vi "读取缺试剂参数.vi"(0 "MB session in":refnum<class "MB_Master.lvclass">, 5 "error in (no error)":errorcluster) -> (14 "MB session out":refnum<class "MB_Master.lvclass">, 15 "评价结果":bool[](array[boolean]), 16 "CH光值":u16[](array[numeric]), 17 "缺试剂类型":u8[](array[numeric]), 18 "光强阈值":u16[](array[numeric]), 19 "error out":errorcluster)   [LabVIEW 2016, in "斯坦道CODMn新电路板.lvlib"]
uses:
  <vilib>/Plasmionique/MB Master/MB_Master/MB_Master.lvclass
  <vilib>/Plasmionique/MB Master/MB_Master_Serial/MB_Master_Serial.lvclass
  D:/Program Files (x86)/National Instruments/LabVIEW 2016/vi.lib/Plasmionique/MB Master/MB_Master/MB_Master.lvclass
  <vilib>/Plasmionique/MB Master/MB Master.lvlib
panel:
  in  "VISA Resource":refnum<visa-resource-name>
  in  "引用选择":enum16{"MB引用", "自建引用"}(ring)
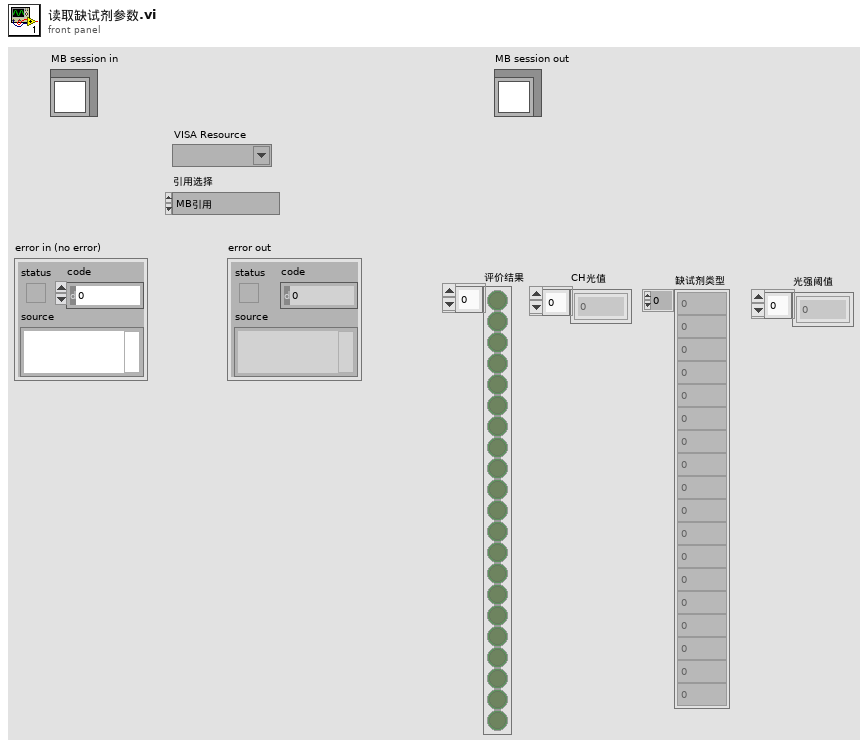
[diagram p1: front panel]
types:
  T1 = cluster{"baud rate (bps)":u32, "stop bits":u16, "parity":u16, "flow control":u16, "timeout":u32, "retries":i32}
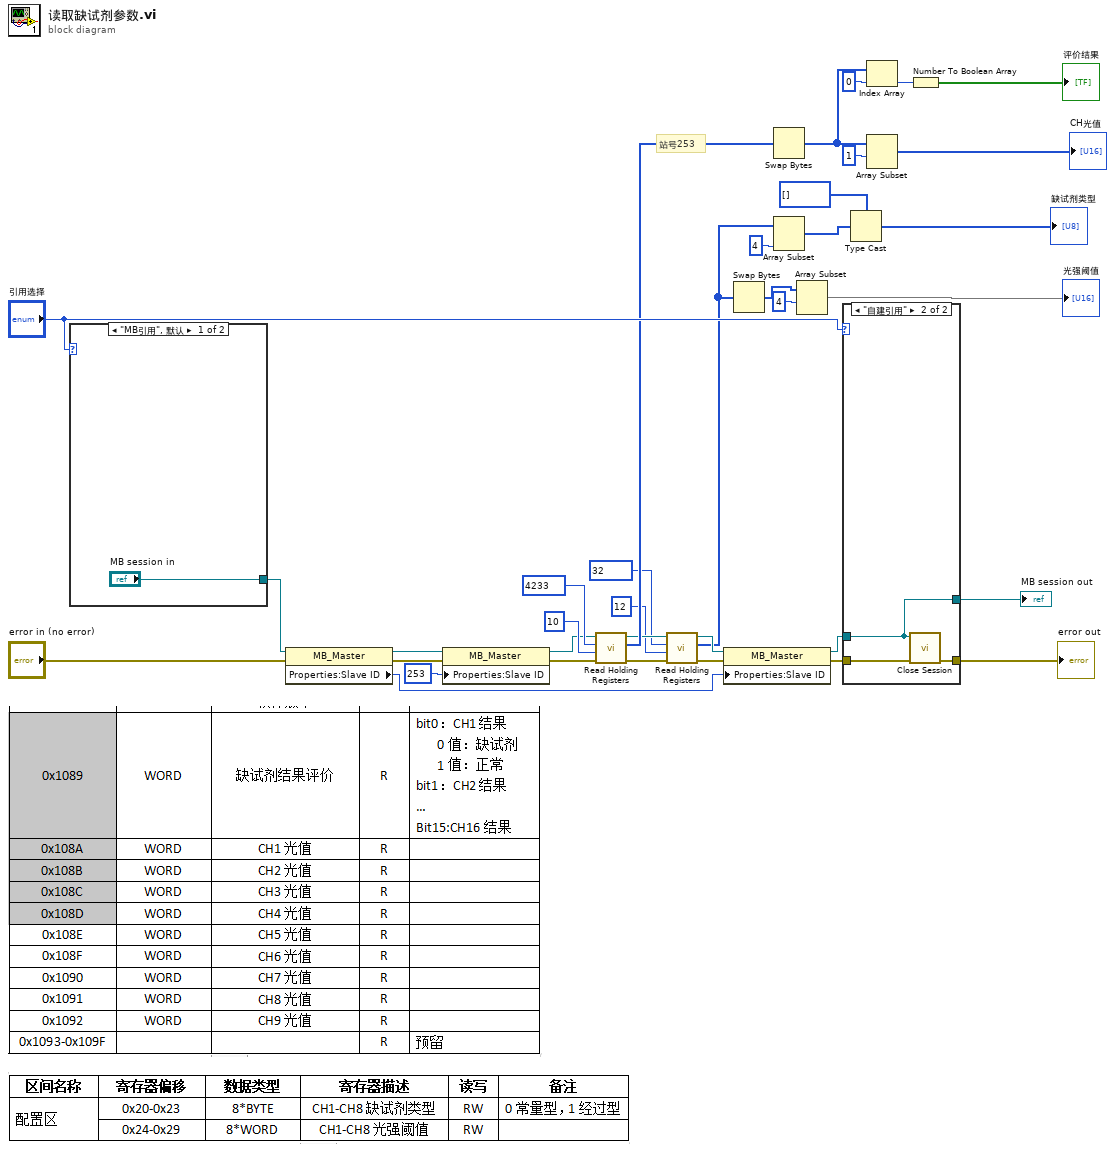
[diagram p0: block diagram]
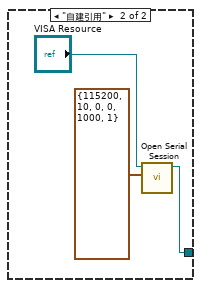
[diagram p3: hidden frame]
diagram:
  # "站号253"
  n1 = case shown="\"MB引用\", 默认" "引用选择" {
    tunnel: ["MB session in" w40] -> w11
    frame "MB引用", Default {
    }
    frame "自建引用" {
      n2 = call <vilib>:"Open Serial Session.vi"("Serial Config"=T1 {"baud rate (bps)"=115200, "stop bits"=10, "parity"=0, "flow control"=0, "timeout"=1000, "retries"=1}, "VISA Resource"="VISA Resource") -> ("MB_Serial session"=w40:refnum<class "MB_Master_Serial.lvclass">)  [unwired: 8 in, 1 out]
    }
  }
  n3 = property class="MB_Master"(reference=w11, error in="error in (no error)") -> (reference out=w9:refnum<class "MB_Master.lvclass">, error out=w8:errorcluster, "Properties:Slave ID"=w3:u8)
  n4 = property class="MB_Master"(reference=w9, error in=w8, "Properties:Slave ID"=u8 253 ("Slave ID")) -> (reference out=w25:refnum<class "MB_Master.lvclass">, error out=w24:errorcluster)
  n5 = call <vilib>:"Read Holding Registers.vi"("error in (no error)"=w24, "quantity"=u16 10, "starting address"=u16 4233, "MB session in"=w25) -> ("error out"=w27:errorcluster, "Registers"=w31:u16[], "MB session out"=w28:refnum<class "MB_Master.lvclass">)  [unwired: 5 in]
  n6 = call <vilib>:"Read Holding Registers.vi"("error in (no error)"=w27, "quantity"=u16 12, "starting address"=u16 32, "MB session in"=w28) -> ("error out"=w6:errorcluster, "Registers"=w2:u16[], "MB session out"=w7:refnum<class "MB_Master.lvclass">)  [unwired: 5 in]
  n7 = property class="MB_Master"(reference=w7, error in=w6, "Properties:Slave ID"=w3) -> (reference out=w5:refnum<class "MB_Master.lvclass">, error out=w4:errorcluster)
  n8 = Swap Bytes(anything=w2) -> (byte swapped=w1:u16[])
  n9 = Swap Bytes(anything=w31) -> (byte swapped=w21:u16[])
  n10 = Array Subset(array=w2, length=4 ("长度")) -> (w17:u16[])  [unwired: 1 in]
  n11 = Array Subset(array=w1, index=4 ("索引")) -> (→"光强阈值":u16[])  [unwired: 1 in]
  n12 = case shown="\"自建引用\"" "引用选择" {
    tunnel: w5 -> [w41 w43]
    tunnel: w4 -> [w42 w45]
    tunnel: [w42 w44] -> w33
    tunnel: [w41 w43] -> w32
    frame "MB引用", Default {
    }
    frame "自建引用" {
      n13 = call-dynamic "Close Session.vi"("error in (no error)"=w45, "MB session in"=w43) -> ("error out"=w44:errorcluster)  [unwired: 9 in]
    }
  }
  "MB session out" <- w32
  "error out" <- w33
  n14 = Type Cast(type=u8[] [], x=w17) -> (*(type *) &x=→"缺试剂类型":u8[])
  n15 = Index Array(array=w21, index=0 ("索引")) -> (element=w20:u16)
  n16 = Array Subset(array=w21, index=1 ("索引")) -> (→"CH光值":u16[])  [unwired: 1 in]
  n17 = Number To Boolean Array(number=w20) -> (Boolean array=→"评价结果":bool[])
